vi "Configure Distance Sensors.vi"(0 "Device ID":T1(ring), 1 "D1_Tolerance":u32=20, 2 "Distance Sensor Mode":enum32{"Voltage", "Distance"}(ring)=enum."Distance", 5 "D1_Level":u32=512, 7 "D1_Repetition_Value":u32=3, 9 "D2_Tolerance":u32=20, 11 "error in":errorcluster, 12 "D2_Level":u32=512, 13 "D2_Repetition_Value":u32=3) -> (4 "Device ID Out":T1(ring), 15 "error out":errorcluster)   [LabVIEW 2010]
doc: "This VI configures the digital distance sensors for the selected Device ID. Currently, the Robo Interface is the only Interface Type to support digital distance sensors."
uses:
  Robo Interface.dll
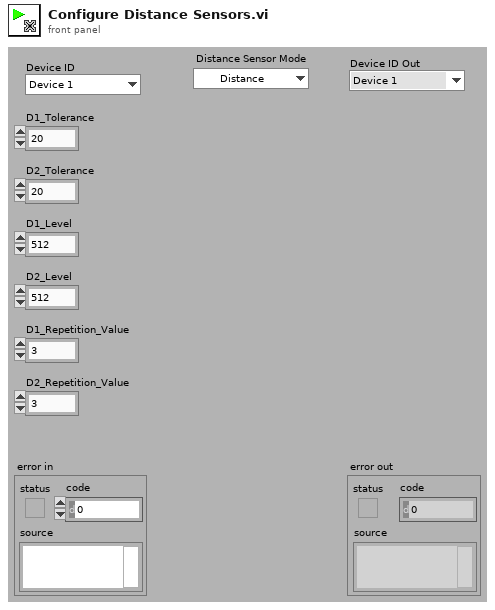
[diagram p1: front panel]
types:
  T1 = enum16{"Device 1", "Device 2", "Device 3", "Device 4", "Device 5", "Device 6", "Device 7", "Device 8"}
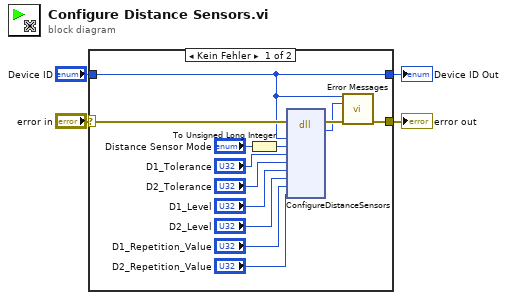
[diagram p0: block diagram]
diagram:
  n1 = case shown="Kein Fehler" "error in" {
    selector: "error in" -> [w16 w19]
    tunnel: [w15 w19] -> w3
    tunnel: "Device ID" -> [w5 w18]
    tunnel: [w5 w18] -> w1
    frame No Error {
      n2 = To Unsigned Long Integer(number="Distance Sensor Mode") -> (unsigned 32bit integer=w13:u32)
      n3 = dll-call lib="D:/Aron/LabVIEW-Programmierung/a.F.b.u.s.A/robo_interface_distribute/Robo Interface/Advanced/Robo Interface.dll" fn="ConfigureDistanceSensors"(error in=w16, "Device_ID"=w5, "Mode"=w13, "D1_Tolerance"="D1_Tolerance", "D2_Tolerance"="D2_Tolerance", "D1_Level"="D1_Level", "D2_Level"="D2_Level", "D1_Repetition_Value"="D1_Repetition_Value", "D2_Repetition_Value"="D2_Repetition_Value") -> (error out=w17:errorcluster, "return type"=w6:i32)  [unwired: 9 in, 2 out]
      n4 = call "Error Messages.vi"("Device ID"=w5, "Error Code"=w6, "error in (no error)"=w17) -> ("error out"=w15:errorcluster)  [unwired: 12 out]
    }
    frame Error {
    }
  }
  "error out" <- w3
  "Device ID Out" <- w1
